vi "close.vi"(8 "error in (no error)":errorcluster, 11 "camera in":refnum<class "camera.lvclass">) -> (0 "error out":errorcluster, 3 "camera out":refnum<class "camera.lvclass">)   [LabVIEW 2017, in "camera.lvclass"]
uses:
  camera.lvclass
  <vilib>/vision/driver/NI_Vision_Acquisition_Software.lvlib
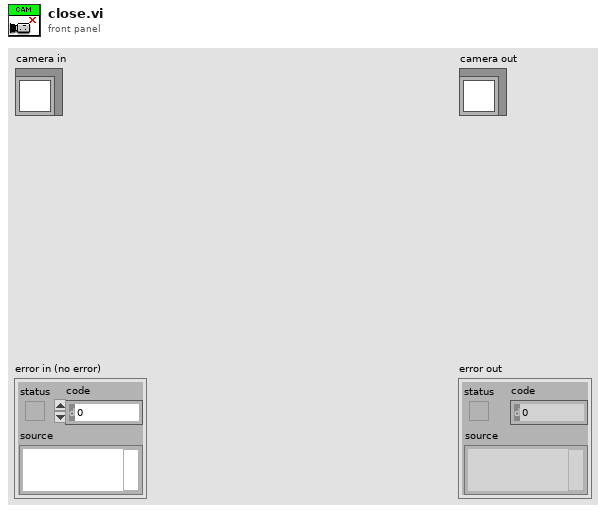
[diagram p1: front panel]
types:
  T1 = typedef "IMAQ Image.ctl" = refnum<image>
  T2 = typedef "IMAQdx.ctl" = refnum<k21>
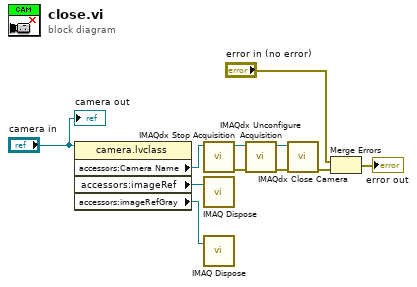
[diagram p0: block diagram]
diagram:
  n1 = property class="camera.lvclass"(reference="camera in") -> ("accessors:Camera Name"=w7:refnum<k21>, "accessors:imageRef"=w5:T1, "accessors:imageRefGray"=w4:T1)  [unwired: 1 in, 2 out]
  n2 = call <vilib>:"IMAQdx Stop Acquisition.vi"("Session In"=w7) -> ("error out"=w8:errorcluster, "Session Out"=w9:T2)  [unwired: 1 in, 8 out]
  n3 = call "IMAQ Dispose"("Image"=w5) -> ()  [unwired: 5 in, 1 out]
  n4 = call "IMAQ Dispose"("Image"=w4) -> ()  [unwired: 5 in, 1 out]
  n5 = call <vilib>:"IMAQdx Unconfigure Acquisition.vi"("error in"=w8, "Session In"=w9) -> ("error out"=w3:errorcluster, "Session Out"=w10:T2)  [unwired: 8 out]
  n6 = call <vilib>:"IMAQdx Close Camera.vi"("error in"=w3, "Session In"=w10) -> ("error out"=w6:errorcluster)  [unwired: 9 out]
  n7 = Merge Errors("error in (no error)", w6) -> (→"error out":errorcluster)
  "camera out" <- "camera in"
